vi "氨氮质控流程.vi"(6 "队列输入NH3":refnum<queue>, 9 "氨氮":bool, 10 "氨氮量程切换":enum32{"H", "L", "AUTO"}(ring)=enum."AUTO") -> (3 "布尔":bool)   [LabVIEW 2016, in "质控单元.lvlib"]
panel:
  out "氨氮中断报警":bool
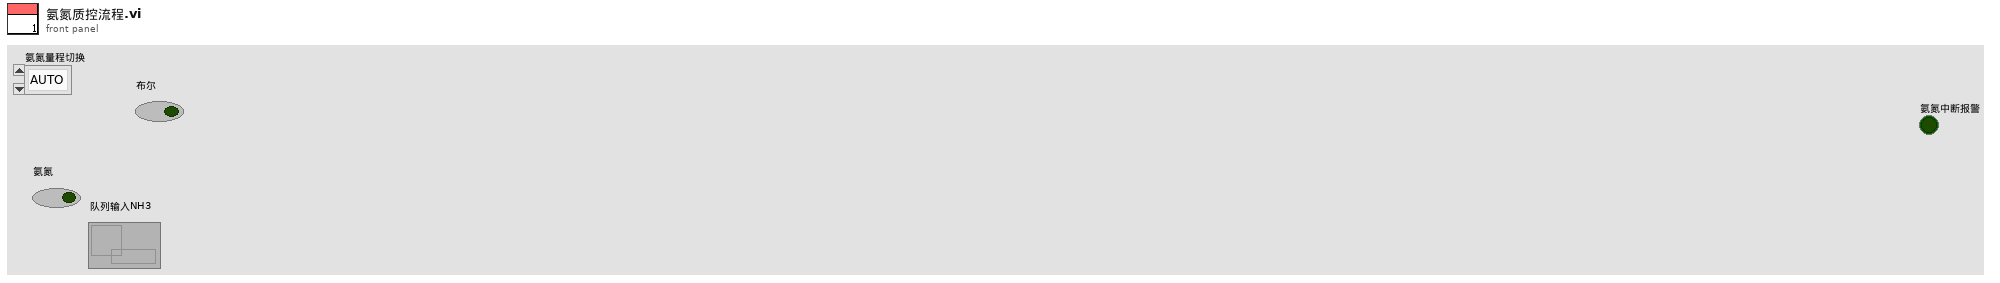
[diagram p1: front panel]
types:
  T1 = enum16{"待机", "启动氨氮水样", "氨氮测量中", "启动氨氮加标", "启动氨氮加标回收", "氨氮加标回收测量中", "启动总氮水样", "总氮测量中", "启动总氮加标", "启动总氮加标回收", "总氮加标回收测量中", "启动总磷水样", "总磷水样测量中", "启动总磷加标", "启动总磷加标回收", "总磷加标回收测量中", "结束"}
  T2 = cluster{"站号":u16, "量程切换":enum32{"H", "L", "AUTO"}, "控制命令":enum16{"启动测量", "标样核查", "零点核查", "跨度核查", "空白测试", "平行样测试", "加标回收", "空白校准", "标样校准", "初始化（清洗）", "停止测试", "仪器重启", "校时", "模式设置", "测量间隔设置"}, "模式设置":enum16{"待机", "连续模式", "周期模式", "定点模式", "受控模式", "手动模式"}, "测量间隔":u16}
  T3 = cluster{"时间标识":timestamp, "设备":string, "日志信息":string}
  T4 = cluster{"系统时间":timestamp, "工作状态":enum16{"空闲", "水样测试", "标样核查", "零点核查", "跨度核查", "空白测试", "平行样测试", "加标回收", "空白校准", "标样校准", "初始化（清洗）"}, "测量模式":enum16{"待机", "连续模式", "周期模式", "定点模式", "受控模式", "手动模式"}, "告警代码":enum16{"无告警", "缺试剂告警", "缺水样告警", "缺蒸馏水告警", "缺标液告警", "仪表漏液告警", "标定异常告警", "超量程告警", "加热异常", "低试剂预警", "超上限告警", "超下限告警", "仪表内部其他异常", "滴定异常告警", "电极异常告警", "量程切换告警", "参数设置告警", "PH电极电位异常", "电导率电极异常", "浊度光度异常", "溶解氧电极异常", "溶解氧光强异常", "温度异常告警", "PH异常告警", "溶解氧异常告警", "电导率异常告警", "浊度异常告警", "叶绿素异常告警", "藻密度异常告警", "蓝绿藻异常告警", "ORP异常告警", "氨氮异常告警", "清洁刷异常告警", "SD卡异常告警", "蓝牙异常告警", "Wifi异常告警", "流程异常告警"}, "故障代码":enum16{"无故障", "电机故障", "温度故障", "通讯故障", "滴定故障"}, "日志代码":u16, "软件版本":u16, "F0":sgl, "F1":sgl, "F2":sgl, "F3":sgl, "T":sgl, "H":sgl, "id":u16, "flowid":u16, "量程":u16, "总磷控温温度1":sgl, "营养盐控温温度2":sgl, "ADC":sgl}
  T5 = enum16{"空闲", "水样测试", "标样核查", "零点核查", "跨度核查", "空白测试", "平行样测试", "加标回收", "空白校准", "标样校准", "初始化（清洗）"}
  T6 = cluster{"因子编码":u32, "单位":u16, "标样参考值":sgl, "水样数据时间":timestamp, "水样实测值":sgl, "水样数据标识":string, "标样数据时间":timestamp, "标样实测值":sgl, "标样数据标识":string, "空白数据时间":timestamp, "空白实测值":sgl, "空白数据标识":string, "零点核查数据时间":timestamp, "零点核查实测值":sgl, "零点核查数据标识":string, "跨度核查数据时间":timestamp, "跨度核查实测值":sgl, "跨度核查数据标识":string, "加标回收数据时间":timestamp, "加标回收实测值":sgl, "加标回收数据标识":string, "平行样数据时间":timestamp, "平行样实测值":sgl, "平行样数据标识":string}
  T7 = cluster{"量程":dbl, "检出限":dbl, "加标前水样浓度":dbl, "加标后水样浓度":dbl, "加标水杯定容体积":dbl, "加标母液浓度":dbl, "加标体积":dbl, "加标回收率":dbl}
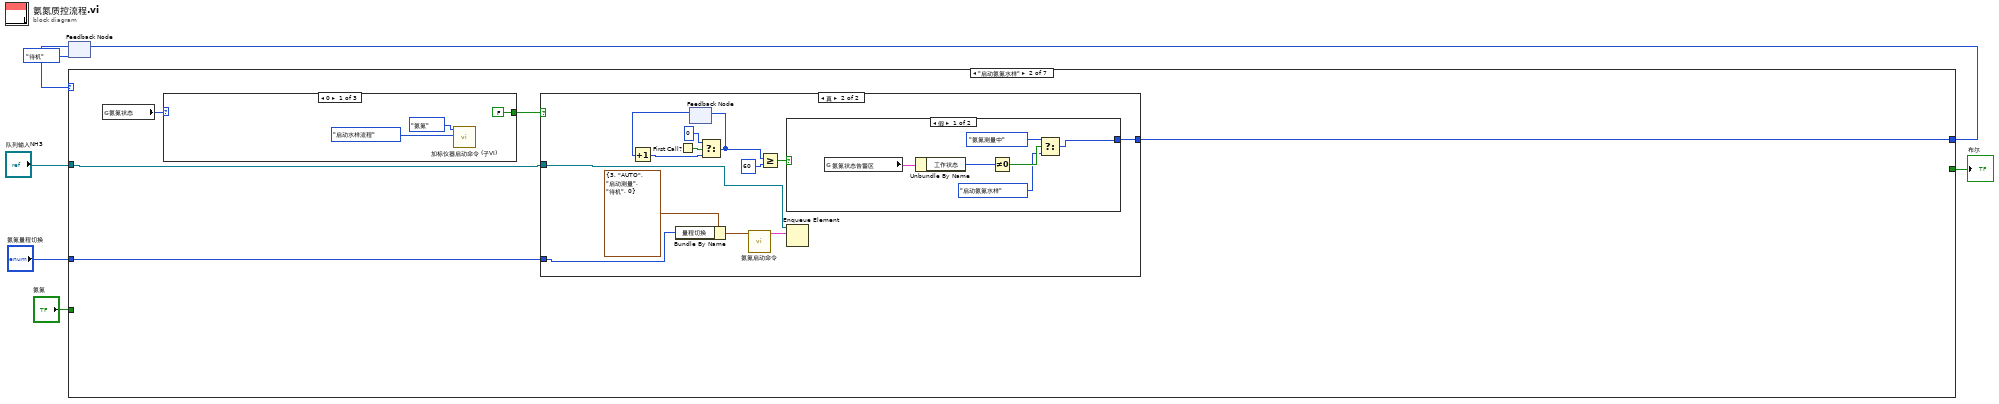
[diagram p0: block diagram]
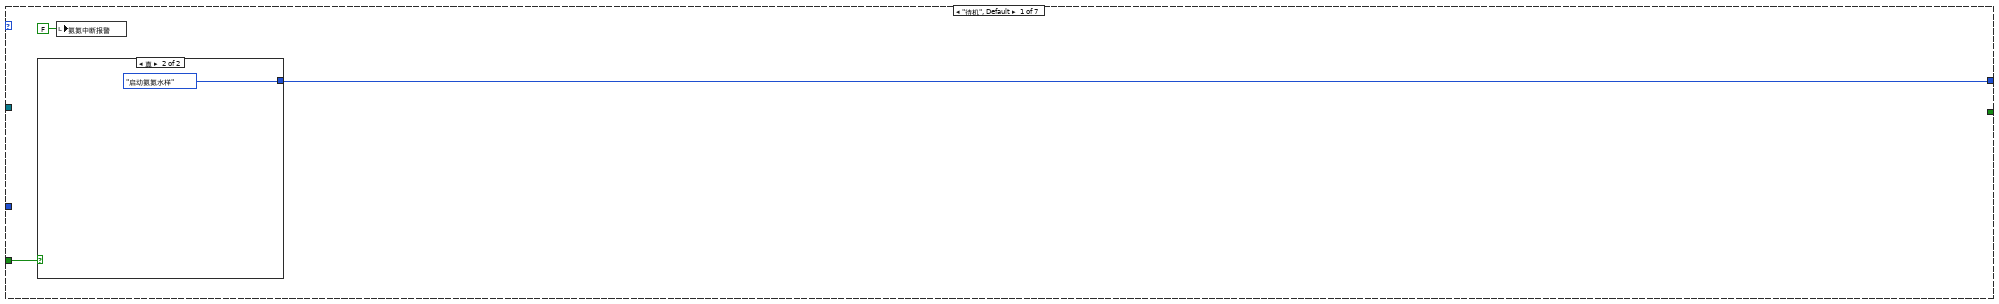
[diagram p2: hidden frame]
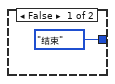
[diagram p3: hidden frame]
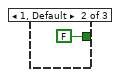
[diagram p4: hidden frame]
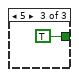
[diagram p5: hidden frame]
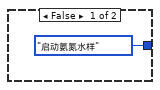
[diagram p6: hidden frame]
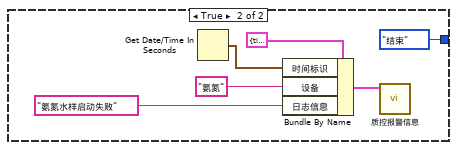
[diagram p7: hidden frame]
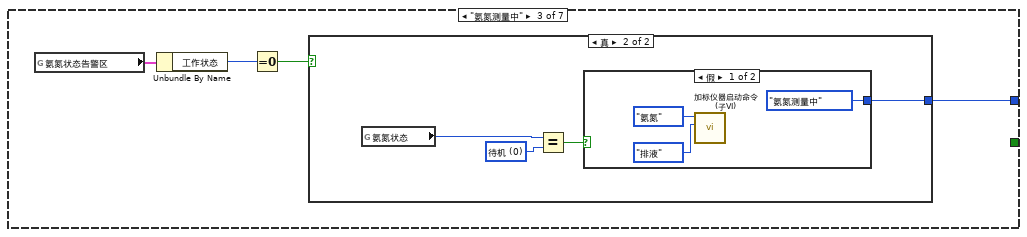
[diagram p8: hidden frame]
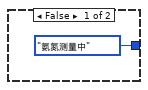
[diagram p9: hidden frame]
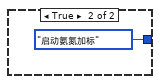
[diagram p10: hidden frame]
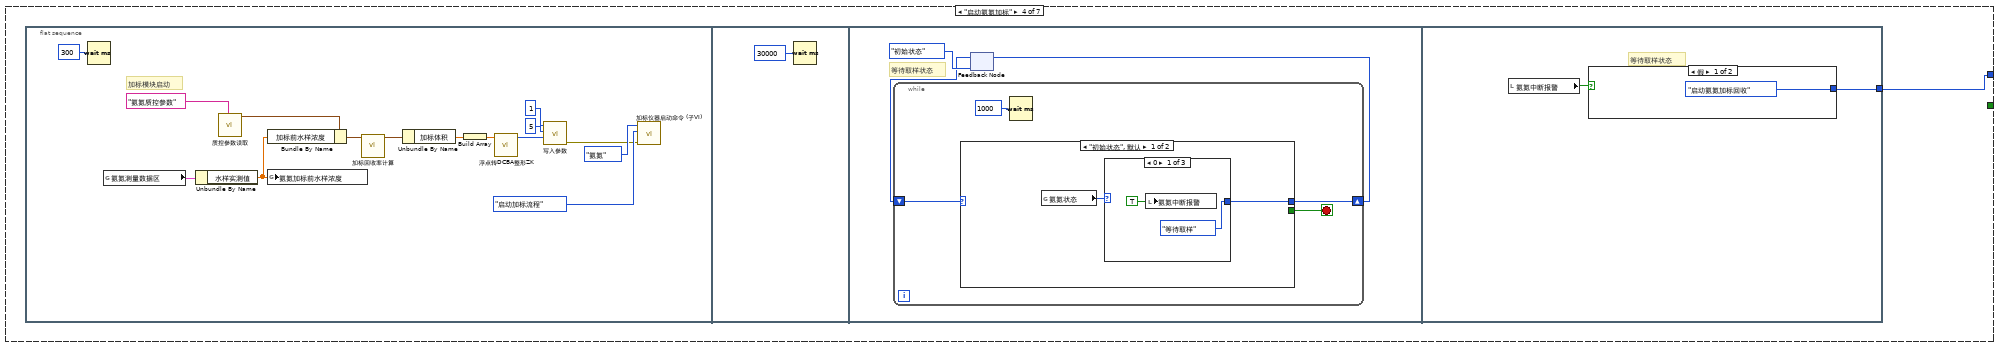
[diagram p11: hidden frame]
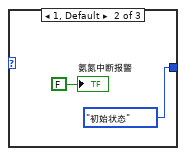
[diagram p12: hidden frame]
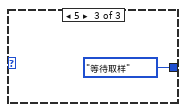
[diagram p13: hidden frame]
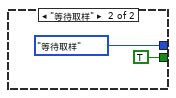
[diagram p14: hidden frame]
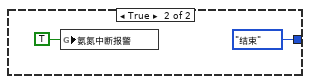
[diagram p15: hidden frame]
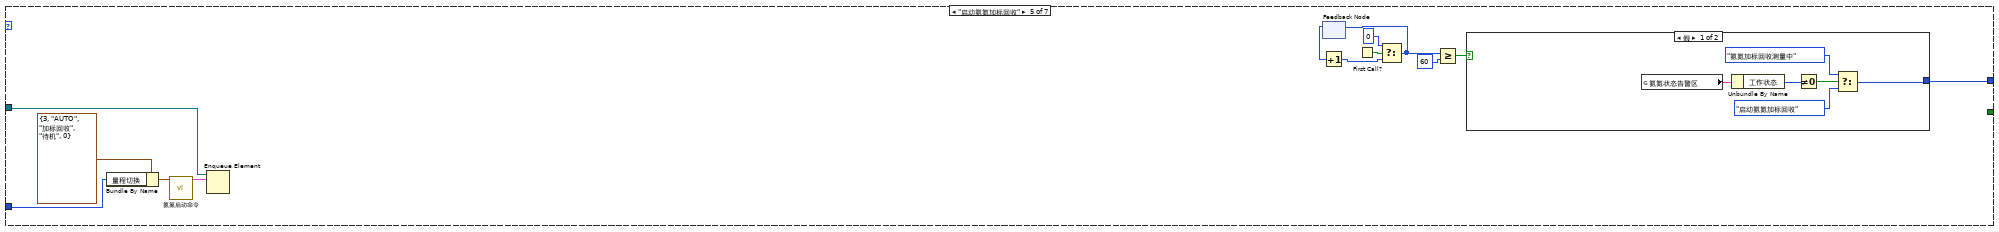
[diagram p16: hidden frame]
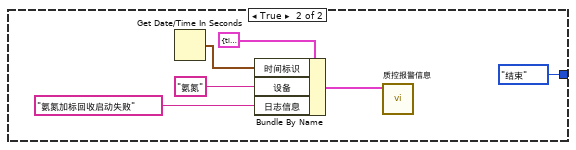
[diagram p17: hidden frame]
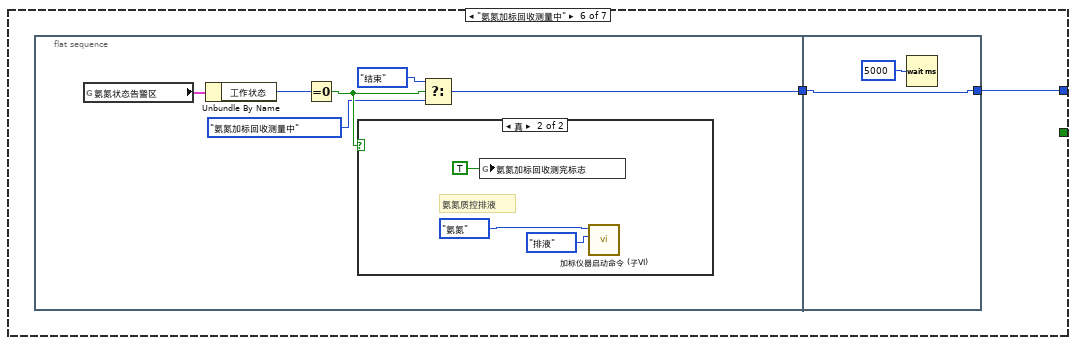
[diagram p18: hidden frame]
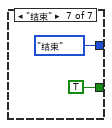
[diagram p20: hidden frame]
diagram:
  n1 = feedback #1(T1."待机") -> (w5:T1)
  n2 = case shown="\"启动氨氮水样\"" w5 {
    tunnel: [w10 w17 w49 w62 w105 w125 T1."结束"] -> w3
    tunnel: [_ _ _ _ _ _ TRUE] -> w6
    tunnel: "氨氮" -> [w9 _ _ _ _ _ _]
    tunnel: "队列输入NH3" -> [_ w16 _ _ w103 _ _]
    tunnel: "氨氮量程切换" -> [_ w15 _ _ w100 _ _]
    frame "待机", Default {
      n3 = case shown="真" w9 {
        tunnel: [T1."结束" T1."启动氨氮水样"] -> w10
        frame False {
        }
        frame True {
        }
      }
      n4 = local write "氨氮中断报警"(FALSE ("氨氮中断报警")) -> ()
    }
    frame "启动氨氮水样" {
      n5 = global read "加标回收状态全局变量.vi" "氨氮状态"() -> (w14:u16)
      n6 = case shown="0" w14 {
        tunnel: [FALSE ("s") FALSE ("s") TRUE ("s")] -> w13
        frame 0 {
          n7 = call "加标仪器启动命令 (子VI).vi"("启动命令"=enum16{"启动水样流程", "启动加标流程", "排液", "停止"}."启动水样流程", "仪器"=enum16{"", "氨氮", "总磷", "总氮", "CODMn", "CODCr"}."氨氮") -> ()  [unwired: 9 in, 1 out]
        }
        frame 1, Default {
        }
        frame 5 {
        }
      }
      n8 = case shown="真" w13 {
        tunnel: [T1."启动氨氮水样" w36] -> w17
        tunnel: w16 -> [_ w27]
        tunnel: w15 -> [_ w24]
        frame False {
        }
        frame True {
          n9 = Bundle By Name(cluster=T2 {"站号"=3, "量程切换"=enum."AUTO", "控制命令"=enum."启动测量", "模式设置"=enum."待机", "测量间隔"=0} ("参数"), "量程切换"=w24) -> (w25:T2)
          n10 = First Call?() -> (First Call?: T/F=w34:bool)
          n11 = feedback #2() -> (w33:i32)  [unwired: 1 in]
          n12 = Increment(x=w33) -> (x+1=w32:i32)
          n13 = Select(t=0, s=w34, f=w32) -> (s? t:f=w31:i32)
          n14 = feedback-in #2(w31) -> ()
          n15 = call "氨氮启动命令.vi"("参数"=w25) -> ("启动命令"=w28:cluster{"命令":string, "data":variant})  [unwired: 10 in]
          n16 = Greater Or Equal?(x=w31, y=60) -> (x >= y?=w29:bool)
          n17 = case shown="假" w29 {
            tunnel: [w40 T1."结束"] -> w36
            frame False {
              n18 = global read "与氨氮交互全局.vi" "氨氮状态告警区"() -> (w37:T4)
              n19 = Unbundle By Name(w37) -> ("工作状态"=w42:T5)
              n20 = Not Equal To 0?(x=w42) -> (x != 0?=w41:bool)
              n21 = Select(t=T1."氨氮测量中", s=w41, f=T1."启动氨氮水样") -> (s? t:f=w40:T1)
            }
            frame True {
              n22 = Get Date/Time In Seconds() -> (seconds since 1Jan1904=w48:timestamp)
              n23 = Bundle By Name(cluster=T3 {"时间标识"=timestamp(0 s since 1904-01-01), "设备"="", "日志信息"=""} ("data in"), "时间标识"=w48, "设备"="氨氮", "日志信息"="氨氮水样启动失败") -> (w43:T3)
              n24 = call "质控报警信息.vi"("data in"=w43) -> ()  [unwired: 10 in, 1 out]
            }
          }
          n25 = Enqueue Element(queue=w27, element=w28) -> ()  [unwired: 2 in, 3 out]
        }
      }
    }
    frame "氨氮测量中" {
      n26 = global read "与氨氮交互全局.vi" "氨氮状态告警区"() -> (w51:T4)
      n27 = Unbundle By Name(w51) -> ("工作状态"=w52:T5)
      n28 = Equal To 0?(x=w52) -> (x = 0?=w50:bool)
      n29 = case shown="真" w50 {
        tunnel: [T1."氨氮测量中" w54] -> w49
        frame False {
        }
        frame True {
          w56 = u16 0 items=["待机", "润洗", "进样", "进样完成", "柱塞泵加标", "等待取液", "排液"] ("氨氮状态")
          n30 = global read "加标回收状态全局变量.vi" "氨氮状态"() -> (w57:u16)
          n31 = Equal?(x=w57, y=w56) -> (x = y?=w55:bool)
          n32 = case shown="假" w55 {
            tunnel: [T1."氨氮测量中" T1."启动氨氮加标"] -> w54
            frame False {
              n33 = call "加标仪器启动命令 (子VI).vi"("启动命令"=enum16{"启动水样流程", "启动加标流程", "排液", "停止"}."排液", "仪器"=enum16{"", "氨氮", "总磷", "总氮", "CODMn", "CODCr"}."氨氮") -> ()  [unwired: 9 in, 1 out]
            }
            frame True {
            }
          }
        }
      }
    }
    frame "启动氨氮加标" {
      n34 = flat-sequence {
        tunnel: [w96] -> w62
        frame #0 {
          # "加标模块启动"
          n35 = Wait (ms)(milliseconds to wait=u32 300 ("等待时间（毫秒）")) -> ()  [unwired: 1 out]
          n36 = global read "与氨氮交互全局.vi" "氨氮测量数据区"() -> (w69:T6)
          n37 = Unbundle By Name(w69) -> ("水样实测值"=w70:sgl)
          n38 = call "质控参数读取.vi"("section"="氨氮质控参数") -> ("参数"=w75:T7)  [unwired: 9 in, 1 out]
          n39 = Bundle By Name(cluster=w75, "加标前水样浓度"=w70) -> (w76:T7)
          n40 = global write "水样浓度全局.vi" "氨氮加标前水样浓度"(w70) -> ()
          n41 = call "加标回收率计算.vi"("参数"=w76) -> ("参数 out"=w74:T7)  [unwired: 10 in]
          n42 = Unbundle By Name(w74) -> ("加标体积"=w71:dbl)
          n43 = Build Array(w71) -> (w67:dbl[])
          n44 = call "浮点转DCBA整形ZK.vi"("浮点数"=w67) -> ("DCBA整形输出"=w66:u16[])  [unwired: 10 in]
          n45 = call "写入参数.vi"("values"=w66, "starting address"=u16 5, "Slave ID"=u16 1 ("value")) -> ("error out"=w63:errorcluster)  [unwired: 8 in]
          n46 = call "加标仪器启动命令 (子VI).vi"("Error in"=w63, "启动命令"=enum16{"启动水样流程", "启动加标流程", "排液", "停止"}."启动加标流程", "仪器"=enum16{"", "氨氮", "总磷", "总氮", "CODMn", "CODCr"}."氨氮") -> ()  [unwired: 8 in, 1 out]
        }
        frame #1 {
          n47 = Wait (ms)(milliseconds to wait=u32 30000 ("等待时间（毫秒）")) -> ()  [unwired: 1 out]
        }
        frame #2 {
          # "等待取样状态"
          n48 = feedback #3(enum16{"初始状态", "等待取样"}."初始状态") -> (w80:enum16{"初始状态", "等待取样"})
          n49 = while {
            shift-right: [w84] -> w79
            shift-left: w80 -> [w85]
            stop <- w83 stop-if-true
            n50 = case shown="\"初始状态\", 默认" w85 {
              tunnel: [w87 enum16{"初始状态", "等待取样"}."等待取样"] -> w84
              tunnel: [_ TRUE] -> w83
              frame "初始状态", Default {
                n51 = global read "加标回收状态全局变量.vi" "氨氮状态"() -> (w86:u16)
                n52 = case shown="0" w86 {
                  tunnel: [enum16{"初始状态", "等待取样"}."等待取样" enum16{"初始状态", "等待取样"}."初始状态" enum16{"初始状态", "等待取样"}."等待取样"] -> w87
                  frame 0 {
                    n53 = local write "氨氮中断报警"(TRUE ("氨氮中断报警")) -> ()
                  }
                  frame 1, Default {
                    "氨氮中断报警" <- FALSE ("总氮中断报警")
                  }
                  frame 5 {
                  }
                }
              }
              frame "等待取样" {
              }
            }
            n54 = Wait (ms)(milliseconds to wait=u32 1000 ("等待时间（毫秒）")) -> ()  [unwired: 1 out]
          }
          n55 = feedback-in #3(w79) -> ()
        }
        frame #3 {
          # "等待取样状态"
          n56 = local read "氨氮中断报警"() -> (w95:bool)
          n57 = case shown="假" w95 {
            tunnel: [T1."启动氨氮加标回收" T1."结束"] -> w96
            frame False {
            }
            frame True {
              n58 = global write "质控中断报警全局.vi" "氨氮中断报警"(TRUE ("氨氮中断报警")) -> ()
            }
          }
        }
      }
    }
    frame "启动氨氮加标回收" {
      n59 = Bundle By Name(cluster=T2 {"站号"=3, "量程切换"=enum."AUTO", "控制命令"=enum."加标回收", "模式设置"=enum."待机", "测量间隔"=0} ("参数"), "量程切换"=w100) -> (w101:T2)
      n60 = call "氨氮启动命令.vi"("参数"=w101) -> ("启动命令"=w104:cluster{"命令":string, "data":variant})  [unwired: 10 in]
      n61 = Enqueue Element(queue=w103, element=w104) -> ()  [unwired: 2 in, 3 out]
      n62 = feedback #4() -> (w110:i32)  [unwired: 1 in]
      n63 = Increment(x=w110) -> (x+1=w109:i32)
      n64 = First Call?() -> (First Call?: T/F=w111:bool)
      n65 = Select(t=0, s=w111, f=w109) -> (s? t:f=w108:i32)
      n66 = feedback-in #4(w108) -> ()
      n67 = Greater Or Equal?(x=w108, y=60) -> (x >= y?=w106:bool)
      n68 = case shown="假" w106 {
        tunnel: [w116 T1."结束"] -> w105
        frame False {
          n69 = global read "与氨氮交互全局.vi" "氨氮状态告警区"() -> (w113:T4)
          n70 = Unbundle By Name(w113) -> ("工作状态"=w118:T5)
          n71 = Not Equal To 0?(x=w118) -> (x != 0?=w117:bool)
          n72 = Select(t=T1."氨氮加标回收测量中", s=w117, f=T1."启动氨氮加标回收") -> (s? t:f=w116:T1)
        }
        frame True {
          n73 = Get Date/Time In Seconds() -> (seconds since 1Jan1904=w124:timestamp)
          n74 = Bundle By Name(cluster=T3 {"时间标识"=timestamp(0 s since 1904-01-01), "设备"="", "日志信息"=""} ("data in"), "时间标识"=w124, "设备"="氨氮", "日志信息"="氨氮加标回收启动失败") -> (w119:T3)
          n75 = call "质控报警信息.vi"("data in"=w119) -> ()  [unwired: 10 in, 1 out]
        }
      }
    }
    frame "氨氮加标回收测量中" {
      n76 = flat-sequence {
        tunnel: [w131] -> w126
        tunnel: [w137] -> w125
        tunnel: w126 -> [w137]
        frame #0 {
          n77 = global read "与氨氮交互全局.vi" "氨氮状态告警区"() -> (w127:T4)
          n78 = Unbundle By Name(w127) -> ("工作状态"=w132:T5)
          n79 = Equal To 0?(x=w132) -> (x = 0?=w129:bool)
          n80 = case shown="真" w129 {
            frame False {
            }
            frame True {
              # "氨氮质控排液"
              n81 = global write "质控测完标志全局 1.vi" "氨氮加标回收测完标志"(TRUE) -> ()
              n82 = call "加标仪器启动命令 (子VI).vi"("启动命令"=enum16{"启动水样流程", "启动加标流程", "排液", "停止"}."排液", "仪器"=enum16{"", "氨氮", "总磷", "总氮", "CODMn", "CODCr"}."氨氮") -> ()  [unwired: 9 in, 1 out]
            }
          }
          n83 = Select(t=T1."结束", s=w129, f=T1."氨氮加标回收测量中") -> (s? t:f=w131:T1)
        }
        frame #1 {
          n84 = Wait (ms)(milliseconds to wait=u32 5000 ("等待时间（毫秒）")) -> ()  [unwired: 1 out]
        }
      }
    }
    frame "结束" {
    }
  }
  "布尔" <- w6
  n85 = feedback-in #1(w3) -> ()
